vi "Parse-element.vi"(8 "error in (no error)":errorcluster, 10 "String in":string, 11 "MarkAbs in":refnum<class "MarkAbs.lvclass">) -> (0 "error out":errorcluster, 1 "Valid element?":bool, 2 "Remaining string":string, 3 "MarkAbs out":refnum<class "MarkAbs.lvclass">)   [LabVIEW 2013, in "MaterialCharacterization.lvlib" / "MarkAbs.lvclass"]
uses:
  MarkAbs.lvclass
  MarkAbs.lvclass/MarkAbs.ctl
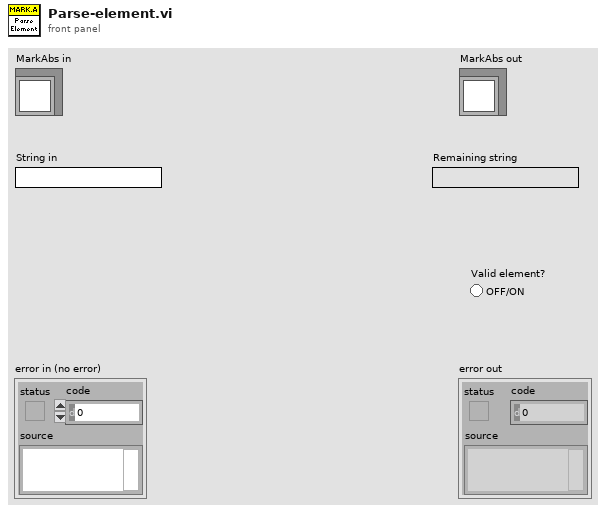
[diagram p1: front panel]
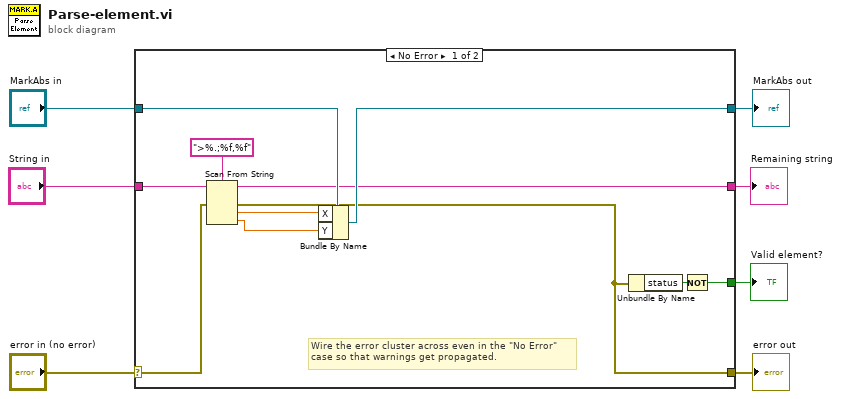
[diagram p0: block diagram]
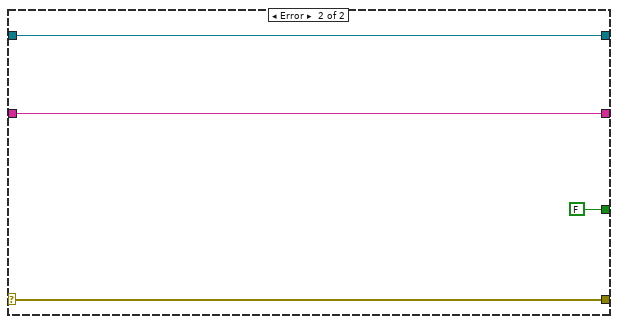
[diagram p2: hidden frame]
diagram:
  n1 = case shown="No Error" "error in (no error)" {
    selector: "error in (no error)" -> [w15 w22]
    tunnel: [w10 w22] -> w6
    tunnel: [w13 w21] -> w4
    tunnel: "MarkAbs in" -> [w14 w21]
    tunnel: "String in" -> [w16 w19]
    tunnel: [w12 w19] -> w2
    tunnel: [w11 FALSE] -> w1
    frame No Error {
      # "Wire the error cluster across even in the \"No Error\"\ncase so that warnings get propagated."
      n2 = Scan From String(format string=">%.;%f,%f", input string=w16, error in=w15) -> (remaining string=w12:string, error out=w10:errorcluster, output 1=w9:dbl, output 2=w8:dbl)  [unwired: 3 in, 1 out]
      n3 = Bundle By Name(cluster=w14, "X"=w9, "Y"=w8) -> (w13:refnum<class "MarkAbs.lvclass">)
      n4 = Unbundle By Name(w10) -> ("status"=w17:bool)
      n5 = Not(x=w17) -> (.not. x?=w11:bool)
    }
    frame Error {
    }
  }
  "error out" <- w6
  "MarkAbs out" <- w4
  "Valid element?" <- w1
  "Remaining string" <- w2
